vi "WS1050_Extract Data From Scope_ST.vi"() -> ()   [LabVIEW 2012]
uses:
  <vilib>/Utility/file.llb/Read From Spreadsheet File (string).vi
panel:
  out "Timming(us)":dbl format="%#_6f"
  out "Time":string[](array[string])
  out "Array 3":string[](array[string])
  out "Amp":string[](array[string])
  out "10% Decrease":string[](array[string])
  out "Numeric 3":dbl
  out "total Runs":i32
  out "Array 2":string[](array[string])
  out "Last Point":dbl
  out "10% Increase":string[](array[string])
  out "all rows":string[][](array[string])
  in  "file path (dialog if empty)":path
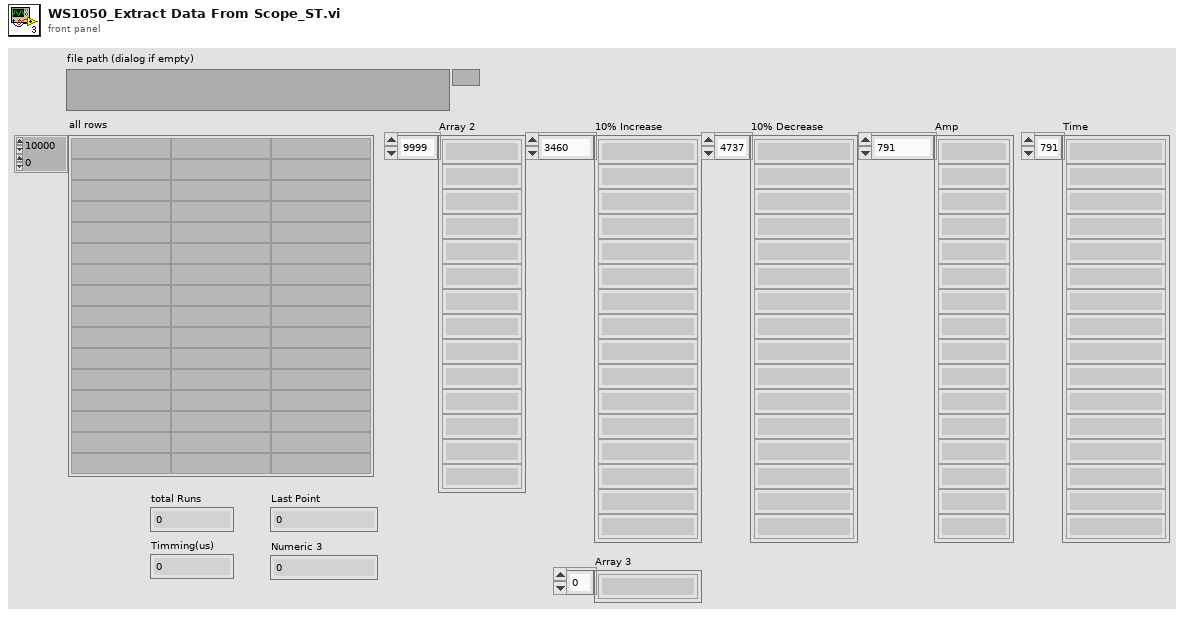
[diagram p1: front panel]
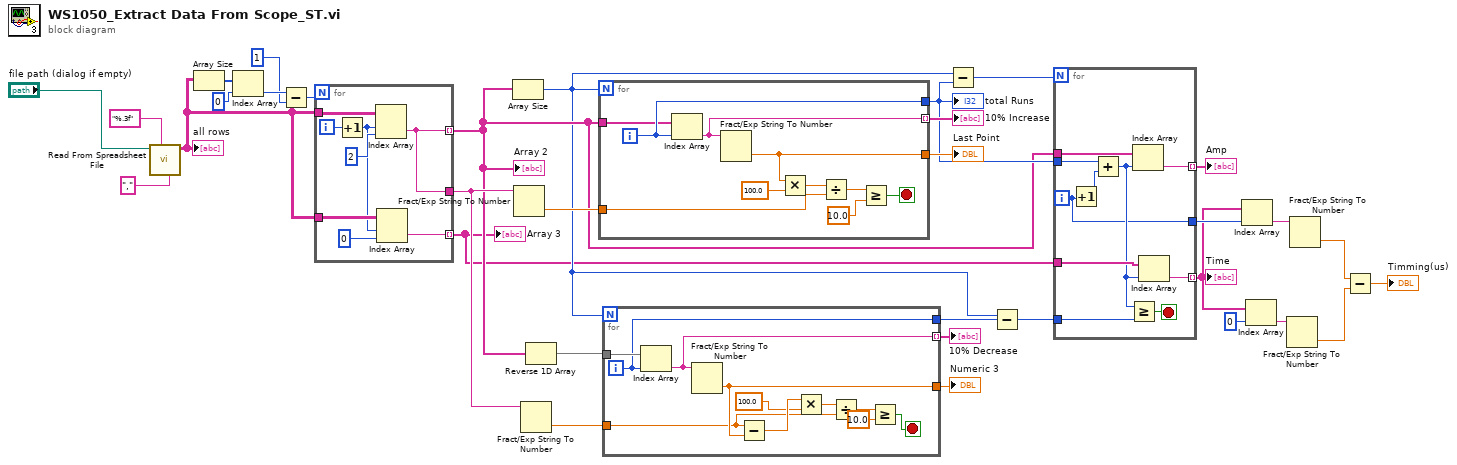
[diagram p0: block diagram]
diagram:
  n1 = call-poly <vilib>:"Read From Spreadsheet File.vi"("delimiter (\\t)"="," ("delimiter (\\t)"), "format (%s)"="%.3f" ("format (%.3f)"), "file path (dialog if empty)"="file path (dialog if empty)") -> ("all rows"=w10:string[][])  [unwired: 4 in, 4 out]
  "all rows" <- w10
  n2 = Array Size(array=w10) -> (size(s)=w30:i32[])
  n3 = Index Array(array=w30, index=0) -> (element=w27:i32)
  n4 = Subtract(x=w27, y=1) -> (x-y=w26:i32)
  n5 = for {
    N: w26 -> [_]
    tunnel: w10 -> [w41]
    tunnel: [w38] -> w14 mode=indexing
    tunnel: [w38] -> w20
    tunnel: w10 -> [w37]
    tunnel: [w34] -> w9 mode=indexing
    i -> [w39]
    n6 = Increment(x=w39) -> (x+1=w36:i32)
    n7 = Index Array(array=w41, index (row)=w36, index (col)=2 ("disabled index (col)")) -> (element=w38:string)
    n8 = Index Array(array=w37, index (row)=w36, index (col)=0 ("disabled index (col)")) -> (element=w34:string)
  }
  "Array 2" <- w14
  "Array 3" <- w9
  n9 = Array Size(array=w14) -> (size(s)=w11:i32)
  n10 = Fract/Exp String To Number(string=w20) -> (number=w28:dbl)  [unwired: 3 in, 1 out]
  n11 = Fract/Exp String To Number(string=w20) -> (number=w24:dbl)  [unwired: 3 in, 1 out]
  n12 = Reverse 1D Array(array=w14) -> (reversed array=w21:string[])
  n13 = for {
    N: w11 -> [_]
    tunnel: w14 -> [w44]
    tunnel: w28 -> [w47]
    tunnel: [w49] -> w19
    tunnel: [w45] -> w17
    tunnel: [w43] -> w18 mode=indexing
    i -> [w45]
    stop <- w42 stop-if-true
    n14 = Index Array(array=w44, index=w45) -> (element=w43:string)
    n15 = Fract/Exp String To Number(string=w43) -> (number=w49:dbl)  [unwired: 3 in, 1 out]
    n16 = Multiply(x=w49, y=100.0) -> (x*y=w48:dbl)
    n17 = Divide(x=w48, y=w47) -> (x/y=w46:dbl)
    n18 = Greater Or Equal?(x=w46, y=10.0) -> (x >= y?=w42:bool)
  }
  "10% Increase" <- w18
  "Last Point" <- w19
  "total Runs" <- w17
  n19 = for {
    N: w11 -> [_]
    tunnel: w21 -> [w62]
    tunnel: w24 -> [w53]
    tunnel: [w56] -> w23
    tunnel: [w57] -> w22 mode=indexing
    tunnel: [w52] -> w12
    i -> [w52]
    stop <- w58 stop-if-true
    n20 = Index Array(array=w62, index=w52) -> (element=w57:string)
    n21 = Fract/Exp String To Number(string=w57) -> (number=w56:dbl)  [unwired: 3 in, 1 out]
    n22 = Subtract(x=w53, y=w56) -> (x-y=w55:dbl)
    n23 = Multiply(x=w55, y=100.0) -> (x*y=w61:dbl)
    n24 = Divide(x=w61, y=w53) -> (x/y=w60:dbl)
    n25 = Greater Or Equal?(x=w60, y=10.0) -> (x >= y?=w58:bool)
  }
  "Numeric 3" <- w23
  "10% Decrease" <- w22
  n26 = Subtract(x=w11, y=w17) -> (x-y=w16:i32)
  n27 = Subtract(x=w11, y=w12) -> (x-y=w13:i32)
  n28 = for {
    N: w16 -> [_]
    tunnel: w17 -> [w72]
    tunnel: w14 -> [w71]
    tunnel: [w70] -> w15 mode=indexing
    tunnel: w13 -> [w68]
    tunnel: w9 -> [w67]
    tunnel: [w66] -> w6 mode=indexing
    tunnel: [w63] -> w8
    i -> [w63]
    stop <- w69 stop-if-true
    n29 = Increment(x=w63) -> (x+1=w64:i32)
    n30 = Add(x=w72, y=w64) -> (x+y=w65:i32)
    n31 = Greater Or Equal?(x=w65, y=w68) -> (x >= y?=w69:bool)
    n32 = Index Array(array=w71, index=w65) -> (element=w70:string)
    n33 = Index Array(array=w67, index=w65) -> (element=w66:string)
  }
  "Amp" <- w15
  "Time" <- w6
  n34 = Index Array(array=w6, index=w8) -> (element=w7:string)
  n35 = Index Array(array=w6, index=0) -> (element=w4:string)
  n36 = Fract/Exp String To Number(string=w4) -> (number=w2:dbl)  [unwired: 3 in, 1 out]
  n37 = Fract/Exp String To Number(string=w7) -> (number=w3:dbl)  [unwired: 3 in, 1 out]
  n38 = Subtract(x=w3, y=w2) -> (x-y=→"Timming(us)":dbl)
